vi "set screen.vi"(0 "VISA in":refnum<visa-resource-name>, 1 "Location Cluster in":T1, 2 "set Screen":string, 5 "error in":errorcluster) -> (14 "VISA out":refnum<visa-resource-name>, 15 "Location Cluster out":T1, 19 "error out":errorcluster)   [LabVIEW 2018]
uses:
  location cluster.ctl
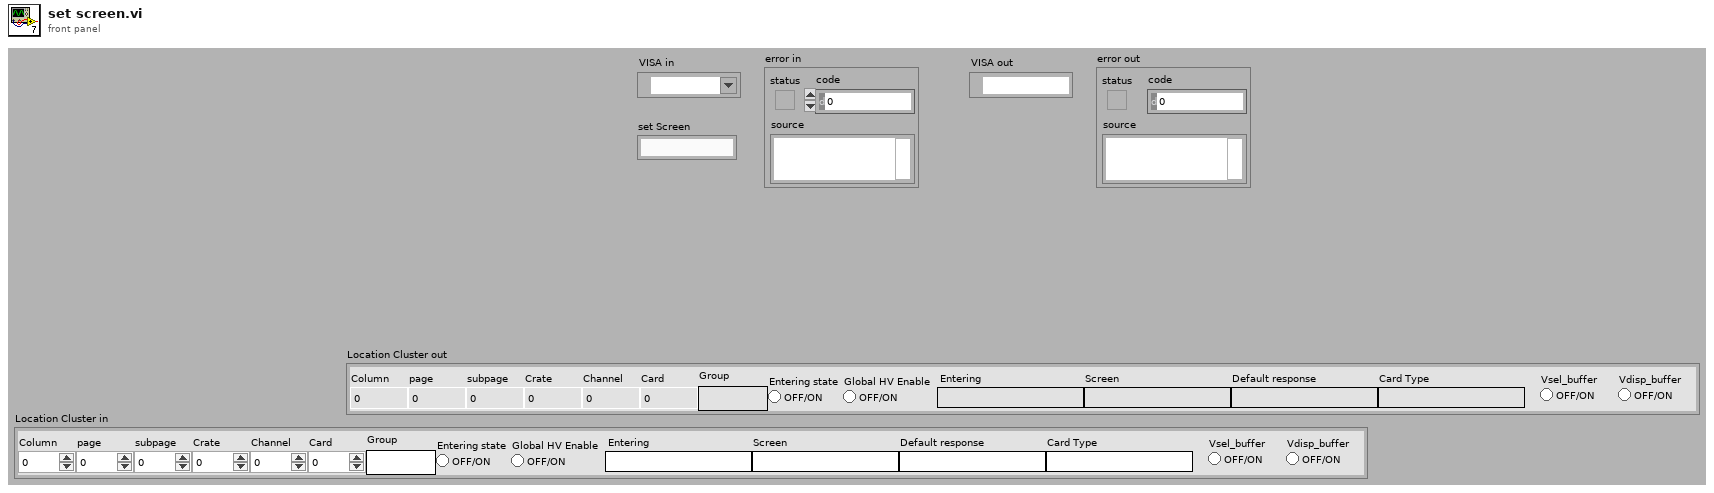
[diagram p1: front panel]
types:
  T1 = typedef "location cluster.ctl" = cluster{"Column":i32, "Card Type":string, "Channel":i32, "Card":i32, "Default response":string, "Entering":string, "Entering state":bool, "subpage":i32, "page":i32, "Crate":i32, "Screen":string, "Group":string, "Global HV Enable":bool, "Vsel_buffer":bool, "Vdisp_buffer":bool}
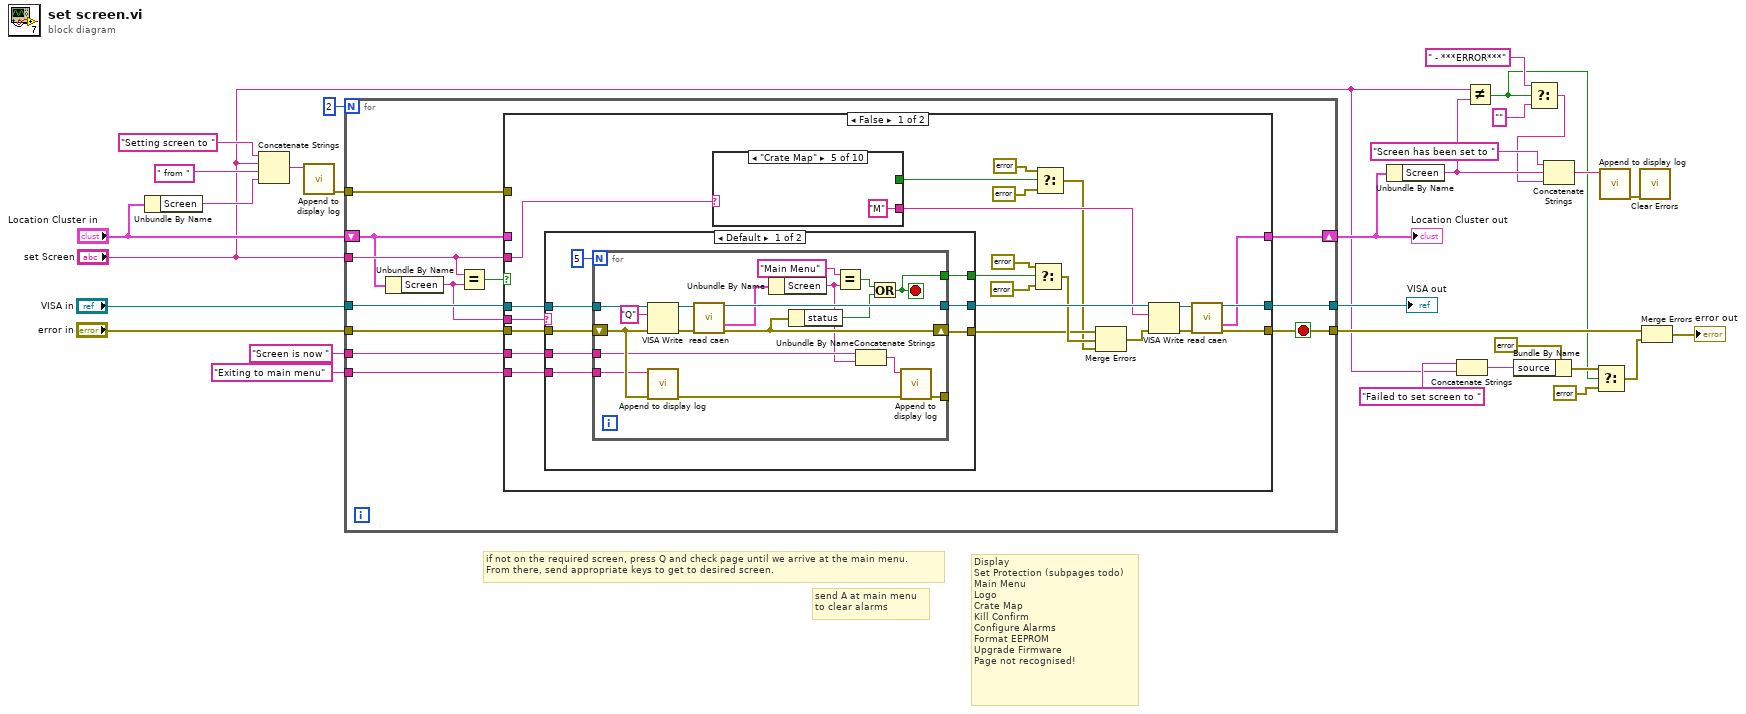
[diagram p0: block diagram]
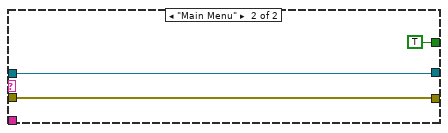
[diagram p2: hidden frame]
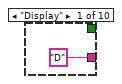
[diagram p3: hidden frame]
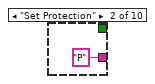
[diagram p4: hidden frame]
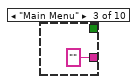
[diagram p5: hidden frame]
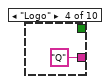
[diagram p6: hidden frame]
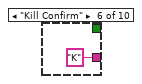
[diagram p7: hidden frame]
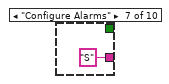
[diagram p8: hidden frame]
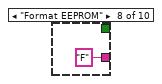
[diagram p9: hidden frame]
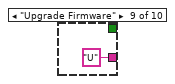
[diagram p10: hidden frame]
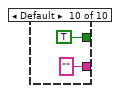
[diagram p11: hidden frame]
diagram:
  # "send A at main menu\nto clear alarms"
  # "Display\nSet Protection (subpages todo)\nMain Menu\nLogo\nCrate Map\nKill Confirm\nConfigure Alarms\nFormat EEPROM\nUpgrade Firmware\nPage not recognised!"
  # "if not on the required screen, press Q and check page until we arrive at the main menu.\nFrom there, send appropriate keys to get to desired screen."
  n1 = Unbundle By Name("Location Cluster in") -> ("Screen"=w21:string)
  n2 = Concatenate Strings("Setting screen to " ("string"), "set Screen", " from " ("string"), w21) -> (w25:string)
  n3 = call "Append to display log.vi"("string"=w25) -> ("error out"=w20:errorcluster)  [unwired: 10 in]
  n4 = for {
    N: 2 -> [_]
    tunnel: w20 -> [w39]
    tunnel: "Exiting to main menu" ("write buffer") -> [w37]
    tunnel: "Screen is now " ("write buffer") -> [w36]
    tunnel: "set Screen" -> [w33]
    shift-right: [w38] -> w19
    shift-left: "Location Cluster in" -> [w32]
    tunnel: "VISA in" -> [w40]
    tunnel: [w42] -> w30
    tunnel: "error in" -> [w41]
    tunnel: [w35] -> w9
    stop <- w35 stop-if-true
    n5 = Unbundle By Name(w32) -> ("Screen"=w31:string)
    n6 = Equal?(x=w33, y=w31) -> (x = y?=w34:bool)
    n7 = case shown="False" w34 {
      tunnel: w40 -> [w65 w107]
      tunnel: w41 -> [w64 w106]
      tunnel: [w57 w107] -> w42
      tunnel: [w58 w106] -> w35
      tunnel: [w56 w108] -> w38
      tunnel: w32 -> [_ w108]
      tunnel: w33 -> [w62 _]
      tunnel: w31 -> [w45 _]
      tunnel: w39 -> [_ _]
      tunnel: w37 -> [w44 _]
      tunnel: w36 -> [w43 _]
      frame False {
        n8 = case shown="Default" w45 {
          tunnel: w65 -> [w73 w94]
          tunnel: w64 -> [w72 w93]
          tunnel: [w70 w94] -> w63
          tunnel: [w69 w93] -> w54
          tunnel: [w68 TRUE] -> w52
          tunnel: w44 -> [w67 _]
          tunnel: w43 -> [w66 _]
          frame Default {
            n9 = for {
              N: 5 -> [_]
              tunnel: w73 -> [w91]
              tunnel: [w88] -> w70
              shift-right: [w87] -> w69
              shift-left: w72 -> [w80]
              tunnel: [w81] -> w68
              tunnel: w67 -> [w79]
              tunnel: w66 -> [w77]
              tunnel: [w74] -> _
              stop <- w81 stop-if-true
              n10 = VISA Write(VISA resource name=w91, write buffer="Q", error in (no error)=w80) -> (VISA resource name out=w90:refnum<visa-resource-name>, error out=w89:errorcluster)  [unwired: 1 out]
              n11 = call "Append to display log.vi"("error in"=w80, "string"=w79) -> ("error out"=w78:errorcluster)  [unwired: 9 in]
              n12 = call "read caen.vi"("VISA in"=w90, "error in"=w89) -> ("VISA out"=w88:refnum<visa-resource-name>, "Location Cluster"=w82:T1, "error out"=w87:errorcluster)  [unwired: 8 in, 3 out]
              n13 = Unbundle By Name(w82) -> ("Screen"=w76:string)
              n14 = Unbundle By Name(w87) -> ("status"=w83:bool)
              n15 = Equal?(x="Main Menu", y=w76) -> (x = y?=w84:bool)
              n16 = Concatenate Strings(w77, w76) -> (w75:string)
              n17 = Or(x=w84, y=w83) -> (x .or. y?=w81:bool)
              n18 = call "Append to display log.vi"("error in"=w78, "string"=w75) -> ("error out"=w74:errorcluster)  [unwired: 9 in]
            }
          }
          frame "Main Menu" {
          }
        }
        n19 = case shown="\"Crate Map\"" w62 {
          tunnel: ["D" ("set Screen") "P" ("set Screen") "" ("set Screen") "Q" ("set Screen") "M" ("set Screen") "K" ("set Screen") "S" ("set Screen") "F" ("set Screen") "U" ("set Screen") "" ("set Screen")] -> w61
          tunnel: [_ _ _ _ _ _ _ _ _ TRUE ("s")] -> w49
          frame "Display" {
          }
          frame "Set Protection" {
          }
          frame "Main Menu" {
          }
          frame "Logo" {
          }
          frame "Crate Map" {
          }
          frame "Kill Confirm" {
          }
          frame "Configure Alarms" {
          }
          frame "Format EEPROM" {
          }
          frame "Upgrade Firmware" {
          }
          frame Default {
          }
        }
        n20 = Select(t=errorcluster {"status"=FALSE, "code"=0, "source"=""} ("f"), s=w52, f=errorcluster {"status"=TRUE, "code"=0, "source"="Did not reach main menu!"} ("input cluster")) -> (s? t:f=w55:errorcluster)
        n21 = Select(t=errorcluster {"status"=TRUE, "code"=0, "source"="Unrecognised Set Page!"} ("input cluster"), s=w49, f=errorcluster {"status"=FALSE, "code"=0, "source"=""}) -> (s? t:f=w48:errorcluster)
        n22 = Merge Errors(w54, w55, w48) -> (w53:errorcluster)
        n23 = VISA Write(VISA resource name=w63, write buffer=w61, error in (no error)=w53) -> (VISA resource name out=w60:refnum<visa-resource-name>, error out=w59:errorcluster)  [unwired: 1 out]
        n24 = call "read caen.vi"("VISA in"=w60, "error in"=w59) -> ("VISA out"=w57:refnum<visa-resource-name>, "Location Cluster"=w56:T1, "error out"=w58:errorcluster)  [unwired: 8 in, 3 out]
      }
      frame True {
      }
    }
  }
  "Location Cluster out" <- w19
  "VISA out" <- w30
  n25 = Unbundle By Name(w19) -> ("Screen"=w13:string)
  n26 = Concatenate Strings("Failed to set screen to " ("string"), "set Screen") -> (w3:string)
  n27 = Not Equal?(x="set Screen", y=w13) -> (x != y?=w4:bool)
  n28 = Bundle By Name(cluster=errorcluster {"status"=TRUE, "code"=0, "source"=""} ("input cluster"), "source"=w3) -> (w5:errorcluster)
  n29 = Select(t=" - ***ERROR***" ("string"), s=w4, f="" ("string")) -> (s? t:f=w12:string)
  n30 = Concatenate Strings("Screen has been set to " ("string"), w13, w12) -> (w24:string)
  n31 = Select(t=w5, s=w4, f=errorcluster {"status"=FALSE, "code"=0, "source"=""}) -> (s? t:f=w7:errorcluster)
  n32 = call "Append to display log.vi"("string"=w24) -> ("error out"=w18:errorcluster)  [unwired: 10 in]
  n33 = call <vilib>:"Clear Errors.vi"("error in (no error)"=w18) -> ()  [unwired: 5 in, 2 out]
  n34 = Merge Errors(w9, w7) -> (→"error out":errorcluster)
